vi "SeCrTs-RD NS Data.vi"(8 "data out":T1, 9 "Array":refnum<queue>[](array[refnum]), 11 "Queue in":refnum<queue>) -> ()   [LabVIEW 2022 SP3]
panel:
  out "overflow? 11":bool
  out "overflow? 10":bool
  out "overflow? 9":bool
  out "overflow? 8":bool
  out "overflow? 7":bool
  out "overflow? 6":bool
  out "overflow? 5":bool
  out "overflow? 4":bool
  out "overflow? 3":bool
  out "overflow? 2":bool
  out "overflow?":bool
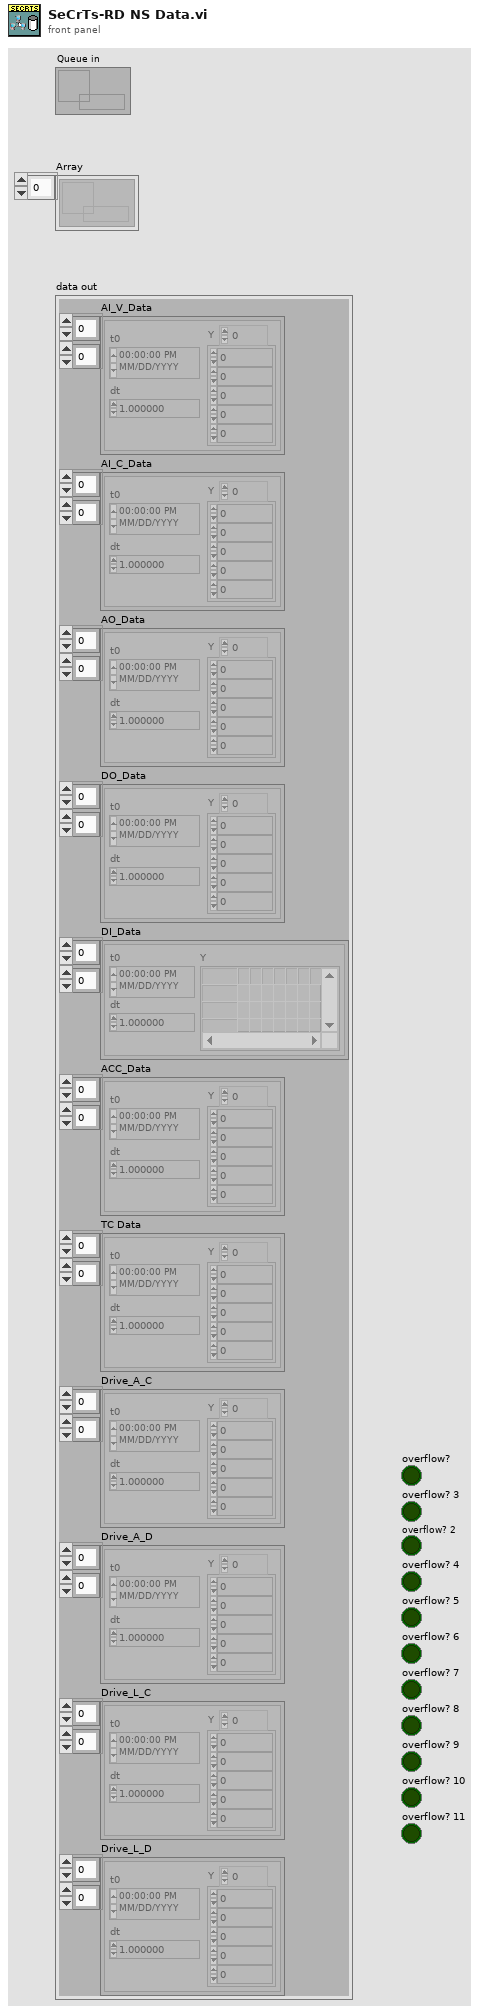
[diagram p1: front panel]
types:
  T1 = cluster{"AI_V_Data":waveform(dbl)[][], "AI_C_Data":waveform(dbl)[][], "AO_Data":waveform(dbl)[][], "DO_Data":waveform(dbl)[][], "DI_Data":digitalwaveform[][], "ACC_Data":waveform(dbl)[][], "TC Data":waveform(dbl)[][], "Drive_A_C":waveform(dbl)[][], "Drive_A_D":waveform(dbl)[][], "Drive_L_C":waveform(dbl)[][], "Drive_L_D":waveform(dbl)[][]}
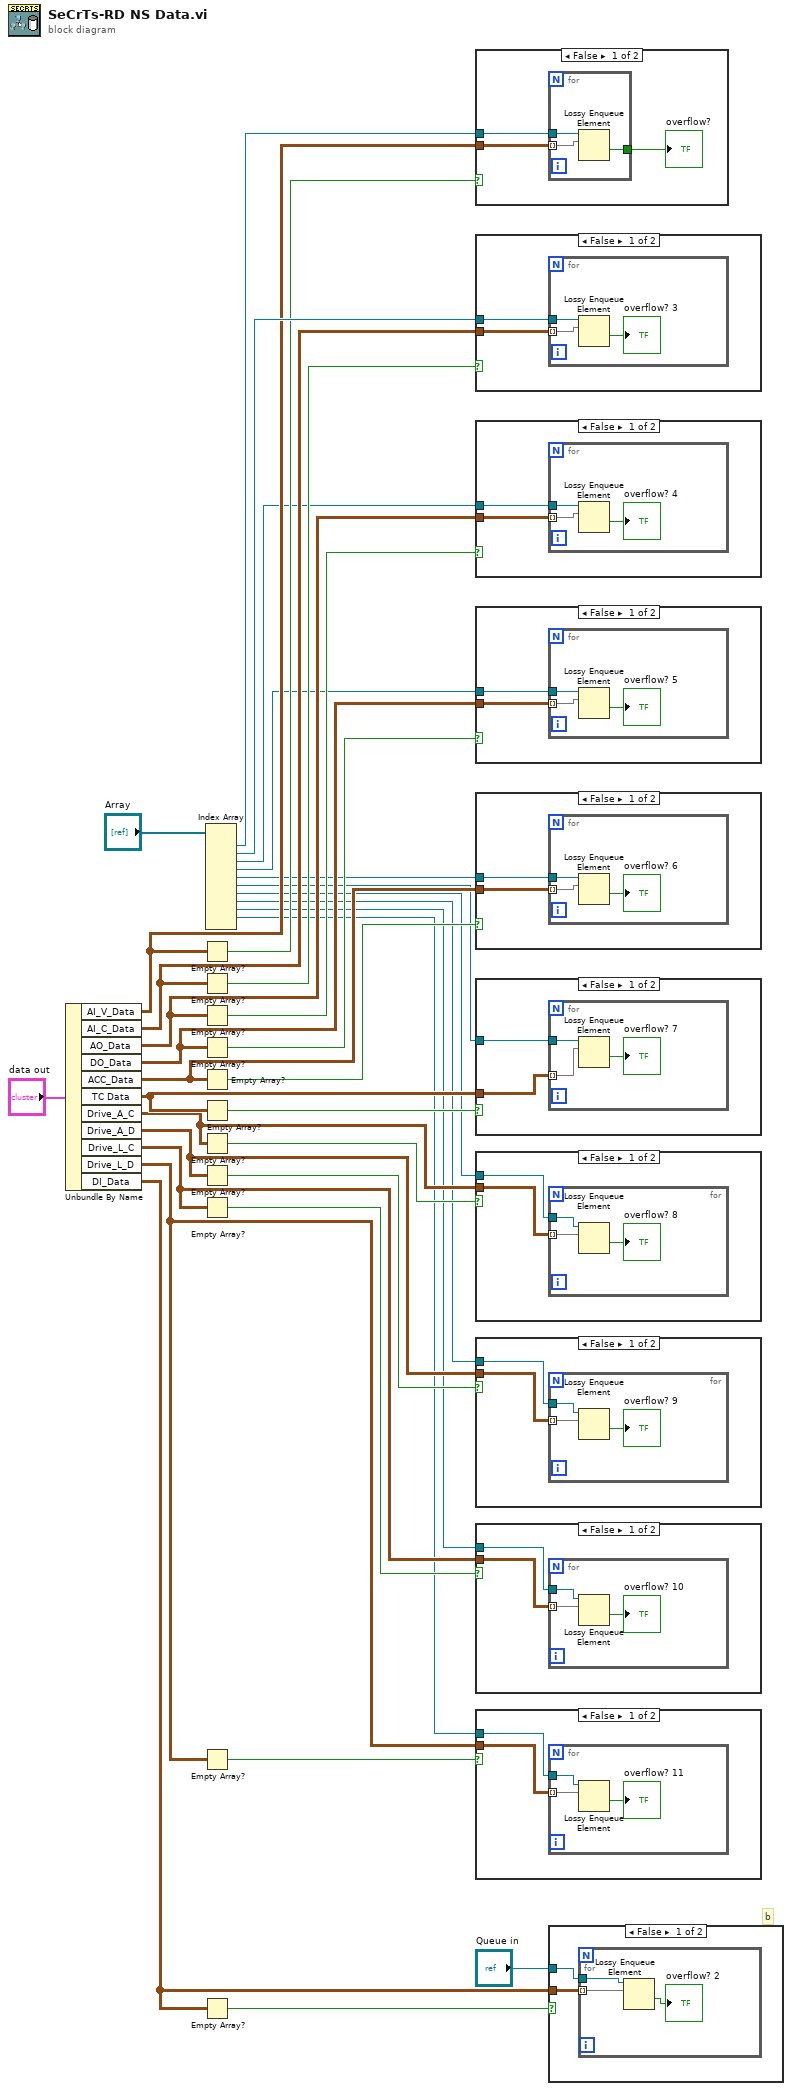
[diagram p0: block diagram]
diagram:
  # "b"
  n1 = Unbundle By Name("data out") -> ("AI_V_Data"=w26:waveform(dbl)[][], "AI_C_Data"=w28:waveform(dbl)[][], "AO_Data"=w22:waveform(dbl)[][], "DO_Data"=w19:waveform(dbl)[][], "ACC_Data"=w17:waveform(dbl)[][], "TC Data"=w14:waveform(dbl)[][], "Drive_A_C"=w11:waveform(dbl)[][], "Drive_A_D"=w8:waveform(dbl)[][], "Drive_L_C"=w6:waveform(dbl)[][], "Drive_L_D"=w2:waveform(dbl)[][], "DI_Data"=w30:digitalwaveform[][])
  n2 = Empty Array?(array=w26) -> (empty?=w27:bool)
  n3 = Empty Array?(array=w28) -> (empty?=w29:bool)
  n4 = Empty Array?(array=w22) -> (empty?=w24:bool)
  n5 = Empty Array?(array=w19) -> (empty?=w21:bool)
  n6 = Empty Array?(array=w17) -> (empty?=w16:bool)
  n7 = Empty Array?(array=w14) -> (empty?=w13:bool)
  n8 = Empty Array?(array=w11) -> (empty?=w10:bool)
  n9 = Empty Array?(array=w8) -> (empty?=w7:bool)
  n10 = Empty Array?(array=w6) -> (empty?=w4:bool)
  n11 = Empty Array?(array=w2) -> (empty?=w1:bool)
  n12 = Empty Array?(array=w30) -> (empty?=w31:bool)
  n13 = Index Array(array="Array") -> (element #1=w33:refnum<queue>, element #2=w34:refnum<queue>, element #3=w23:refnum<queue>, element #4=w20:refnum<queue>, element #5=w18:refnum<queue>, element #6=w15:refnum<queue>, element #7=w12:refnum<queue>, element #8=w9:refnum<queue>, element #9=w5:refnum<queue>, element #10=w3:refnum<queue>)  [unwired: 11 in, 1 out]
  n14 = case shown="False" w27 {
    tunnel: w26 -> [w38 _]
    tunnel: w33 -> [w37 _]
    frame False {
      n15 = for {
        tunnel: w38 -> [w39] mode=indexing
        tunnel: w37 -> [w41]
        tunnel: [w40] -> w36
        n16 = Lossy Enqueue Element(queue=w41, element=w39) -> (overflow?=w40:bool)  [unwired: 1 in, 3 out]
      }
      "overflow?" <- w36
    }
    frame True {
    }
  }
  n17 = case shown="False" w29 {
    tunnel: w28 -> [w43 _]
    tunnel: w34 -> [w42 _]
    frame False {
      n18 = for {
        tunnel: w43 -> [w46] mode=indexing
        tunnel: w42 -> [w45]
        n19 = Lossy Enqueue Element(queue=w45, element=w46) -> (overflow?=→"overflow? 3":bool)  [unwired: 1 in, 3 out]
      }
    }
    frame True {
    }
  }
  n20 = case shown="False" w24 {
    tunnel: w22 -> [w48 _]
    tunnel: w23 -> [w47 _]
    frame False {
      n21 = for {
        tunnel: w48 -> [w51] mode=indexing
        tunnel: w47 -> [w50]
        n22 = Lossy Enqueue Element(queue=w50, element=w51) -> (overflow?=→"overflow? 4":bool)  [unwired: 1 in, 3 out]
      }
    }
    frame True {
    }
  }
  n23 = case shown="False" w21 {
    tunnel: w19 -> [w53 _]
    tunnel: w20 -> [w52 _]
    frame False {
      n24 = for {
        tunnel: w53 -> [w54] mode=indexing
        tunnel: w52 -> [w56]
        n25 = Lossy Enqueue Element(queue=w56, element=w54) -> (overflow?=→"overflow? 5":bool)  [unwired: 1 in, 3 out]
      }
    }
    frame True {
    }
  }
  n26 = case shown="False" w16 {
    tunnel: w17 -> [w58 _]
    tunnel: w18 -> [w57 _]
    frame False {
      n27 = for {
        tunnel: w58 -> [w59] mode=indexing
        tunnel: w57 -> [w61]
        n28 = Lossy Enqueue Element(queue=w61, element=w59) -> (overflow?=→"overflow? 6":bool)  [unwired: 1 in, 3 out]
      }
    }
    frame True {
    }
  }
  n29 = case shown="False" w13 {
    tunnel: w14 -> [w63 _]
    tunnel: w15 -> [w62 _]
    frame False {
      n30 = for {
        tunnel: w63 -> [w64] mode=indexing
        tunnel: w62 -> [w66]
        n31 = Lossy Enqueue Element(queue=w66, element=w64) -> (overflow?=→"overflow? 7":bool)  [unwired: 1 in, 3 out]
      }
    }
    frame True {
    }
  }
  n32 = case shown="False" w10 {
    tunnel: w11 -> [w68 _]
    tunnel: w12 -> [w67 _]
    frame False {
      n33 = for {
        tunnel: w68 -> [w69] mode=indexing
        tunnel: w67 -> [w71]
        n34 = Lossy Enqueue Element(queue=w71, element=w69) -> (overflow?=→"overflow? 8":bool)  [unwired: 1 in, 3 out]
      }
    }
    frame True {
    }
  }
  n35 = case shown="False" w7 {
    tunnel: w8 -> [w73 _]
    tunnel: w9 -> [w72 _]
    frame False {
      n36 = for {
        tunnel: w73 -> [w74] mode=indexing
        tunnel: w72 -> [w76]
        n37 = Lossy Enqueue Element(queue=w76, element=w74) -> (overflow?=→"overflow? 9":bool)  [unwired: 1 in, 3 out]
      }
    }
    frame True {
    }
  }
  n38 = case shown="False" w4 {
    tunnel: w6 -> [w78 _]
    tunnel: w5 -> [w77 _]
    frame False {
      n39 = for {
        tunnel: w78 -> [w79] mode=indexing
        tunnel: w77 -> [w81]
        n40 = Lossy Enqueue Element(queue=w81, element=w79) -> (overflow?=→"overflow? 10":bool)  [unwired: 1 in, 3 out]
      }
    }
    frame True {
    }
  }
  n41 = case shown="False" w1 {
    tunnel: w2 -> [w83 _]
    tunnel: w3 -> [w82 _]
    frame False {
      n42 = for {
        tunnel: w83 -> [w84] mode=indexing
        tunnel: w82 -> [w86]
        n43 = Lossy Enqueue Element(queue=w86, element=w84) -> (overflow?=→"overflow? 11":bool)  [unwired: 1 in, 3 out]
      }
    }
    frame True {
    }
  }
  n44 = case shown="False" w31 {
    tunnel: w30 -> [w88 _]
    tunnel: "Queue in" -> [w87 _]
    frame False {
      n45 = for {
        tunnel: w88 -> [w91] mode=indexing
        tunnel: w87 -> [w90]
        n46 = Lossy Enqueue Element(queue=w90, element=w91) -> (overflow?=→"overflow? 2":bool)  [unwired: 1 in, 3 out]
      }
    }
    frame True {
    }
  }
